vi "Load_Program - copia.vi"(2 "error in (no error)":errorcluster, 3 "FLASH":bool, 4 "Queue in":refnum<queue>) -> (0 "error out":errorcluster, 1 "Queue out":refnum<queue>)   [LabVIEW 2018]
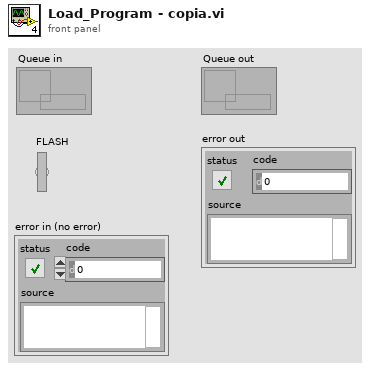
[diagram p1: front panel]
types:
  T1 = enum16{"Write Enable", "Page Program", "Write Disable", "Read Status", "Read Memory"}
  T2 = enum16{"Write Enable", "Page Program", "Write Disable", "Read Status"}
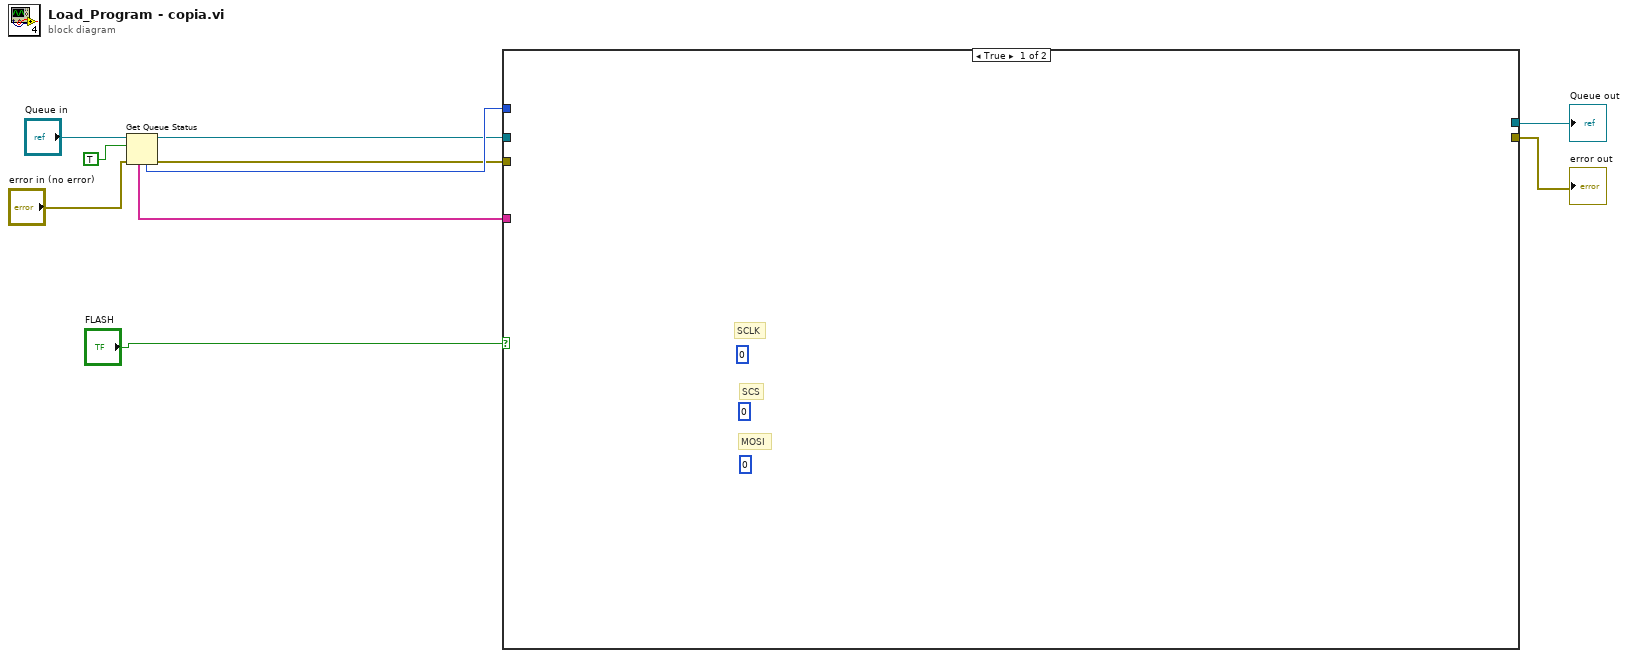
[diagram p0: block diagram]
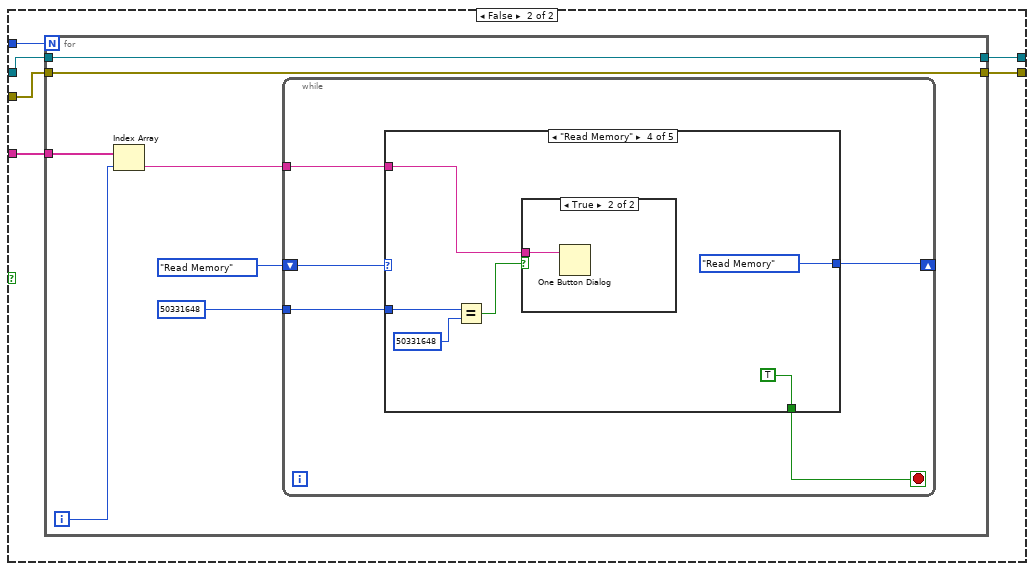
[diagram p2: hidden frame]
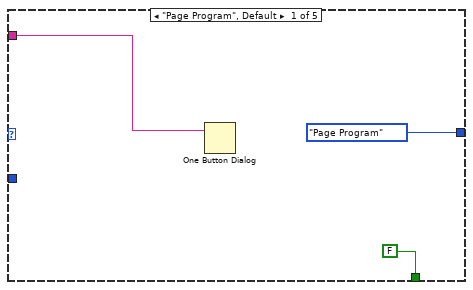
[diagram p3: hidden frame]
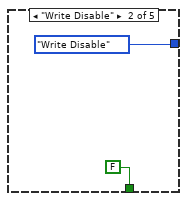
[diagram p4: hidden frame]
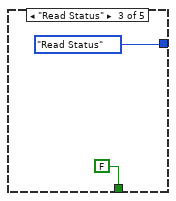
[diagram p5: hidden frame]
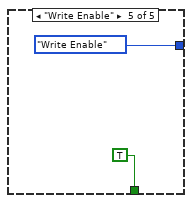
[diagram p7: hidden frame]
diagram:
  n1 = Get Queue Status(queue="Queue in", return elements? (F)=TRUE, error in (no error)="error in (no error)") -> (queue out=w5:refnum<queue>, error out=w3:errorcluster, # elements in queue=w9:i32, elements=w6:string[])  [unwired: 4 out]
  n2 = case shown="True" "FLASH" {
    tunnel: w9 -> [_ w16]
    tunnel: w6 -> [_ w15]
    tunnel: w5 -> [_ w14]
    tunnel: [_ w13] -> w4
    tunnel: w3 -> [_ w12]
    tunnel: [_ w11] -> w2
    frame True {
      (unwired) 0
      (unwired) 0
      (unwired) 0
      # "MOSI"
      # "SCS"
      # "SCLK"
    }
    frame False {
      n3 = for {
        N: w16 -> [_]
        tunnel: w15 -> [w23]
        tunnel: w14 -> [w19]
        tunnel: [w19] -> w13
        tunnel: w12 -> [w18]
        tunnel: [w18] -> w11
        i -> [w22]
        n4 = Index Array(array=w23, index=w22) -> (element=w20:string)
        n5 = while {
          shift-right: [w27] -> _
          shift-left: T1."Read Memory" -> [w28]
          tunnel: w20 -> [w25]
          tunnel: 50331648 -> [w24]
          stop <- w26 stop-if-true
          n6 = case shown="\"Read Memory\"" w28 {
            tunnel: [T2."Page Program" T2."Write Disable" T2."Read Status" T1."Read Memory" T2."Write Enable"] -> w27
            tunnel: [FALSE FALSE FALSE TRUE TRUE] -> w26
            tunnel: w25 -> [w29 _ _ w40 _]
            tunnel: w24 -> [_ _ _ w37 _]
            frame "Page Program", Default {
              n7 = One Button Dialog(message=w29) -> ()  [unwired: 1 in, 1 out]
            }
            frame "Write Disable" {
            }
            frame "Read Status" {
            }
            frame "Read Memory" {
              n8 = Equal?(x=w37, y=50331648) -> (x = y?=w36:bool)
              n9 = case shown="True" w36 {
                tunnel: w40 -> [_ w42]
                frame False {
                }
                frame True {
                  n10 = One Button Dialog(message=w42) -> ()  [unwired: 1 in, 1 out]
                }
              }
            }
            frame "Write Enable" {
            }
          }
        }
      }
    }
  }
  "Queue out" <- w4
  "error out" <- w2
